vi "Insert VI into SubPanel.vi"(9 "error in":errorcluster, 10 "SubPnl Ref":refnum<vi>, 11 "VI in":refnum<vi>) -> (1 "error out":errorcluster)   [LabVIEW 2023, in "Message Queue Helper.lvlib"]
uses:
  Message Queue Helper.lvlib
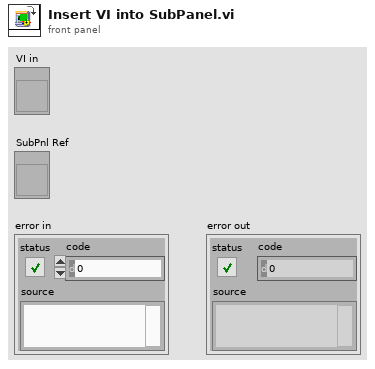
[diagram p1: front panel]
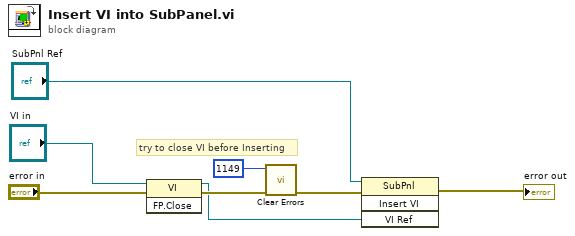
[diagram p0: block diagram]
diagram:
  # "try to close VI before Inserting"
  n1 = invoke class="VI" method="FP.Close"(reference="VI in", error in="error in") -> (reference out=w2:refnum<vi>, error out=w7:errorcluster)  [unwired: 1 in, 1 out]
  n2 = call <vilib>:"Clear Errors.vi"("error in (no error)"=w7, "specific error code to clear (0: all)"=1149) -> ("error out"=w4:errorcluster)  [unwired: 4 in, 1 out]
  n3 = invoke on="Invoke Node" class="SubPnl" method="Insert VI"(reference="SubPnl Ref", error in=w4, "VI Ref"=w2) -> (error out=→"error out":errorcluster)  [unwired: 1 in, 3 out]
